vi "Single point scan V1.vi"() -> ()   [LabVIEW 2024]
uses:
  <vilib>/DAQmx/create/channels.llb/DAQmx Create Channel (AO-Voltage-Basic).vi
  <vilib>/DAQmx/miscellaneous.llb/DAQmx Fill In Error Info.vi
  <vilib>/DAQmx/configure/trigger.llb/DAQmx Start Trigger (None).vi
  <vilib>/DAQmx/configure/timing.llb/DAQmx Timing (Sample Clock).vi
  <vilib>/DAQmx/write.llb/DAQmx Write (Analog 1D DBL NChan 1Samp).vi
  <vilib>/DAQmx/read.llb/DAQmx Read (Analog 1D DBL 1Chan NSamp).vi
  <vilib>/DAQmx/create/channels.llb/DAQmx Create Channel (AI-Voltage-Basic).vi
  <vilib>/vision/driver/NI_Vision_Acquisition_Software.lvlib
panel:
  in  "Camera Name":refnum<k21> caption="IMAQdx Session"
  out "Image":T1(plugin-control)
  out "Filename Out":path
  in  "Filename":path=path "test.lvm"
  in  "Enable data file creation":bool=TRUE caption="Enable"
  out "output waveform":waveform(dbl)
  out "Waveform Graph":dbl[](graph)
  in  "start acquisition":bool
  in  "total samples":i32=1000
  in  "rate (Hz)":dbl=1000.0 format="%0.2f"
  in  "Y-axis":dbl(slide) scale=-10.0..10.0
  in  "X-axis":dbl(slide) scale=-10.0..10.0
  # "Data settings"
  # "Adjust Laser position"
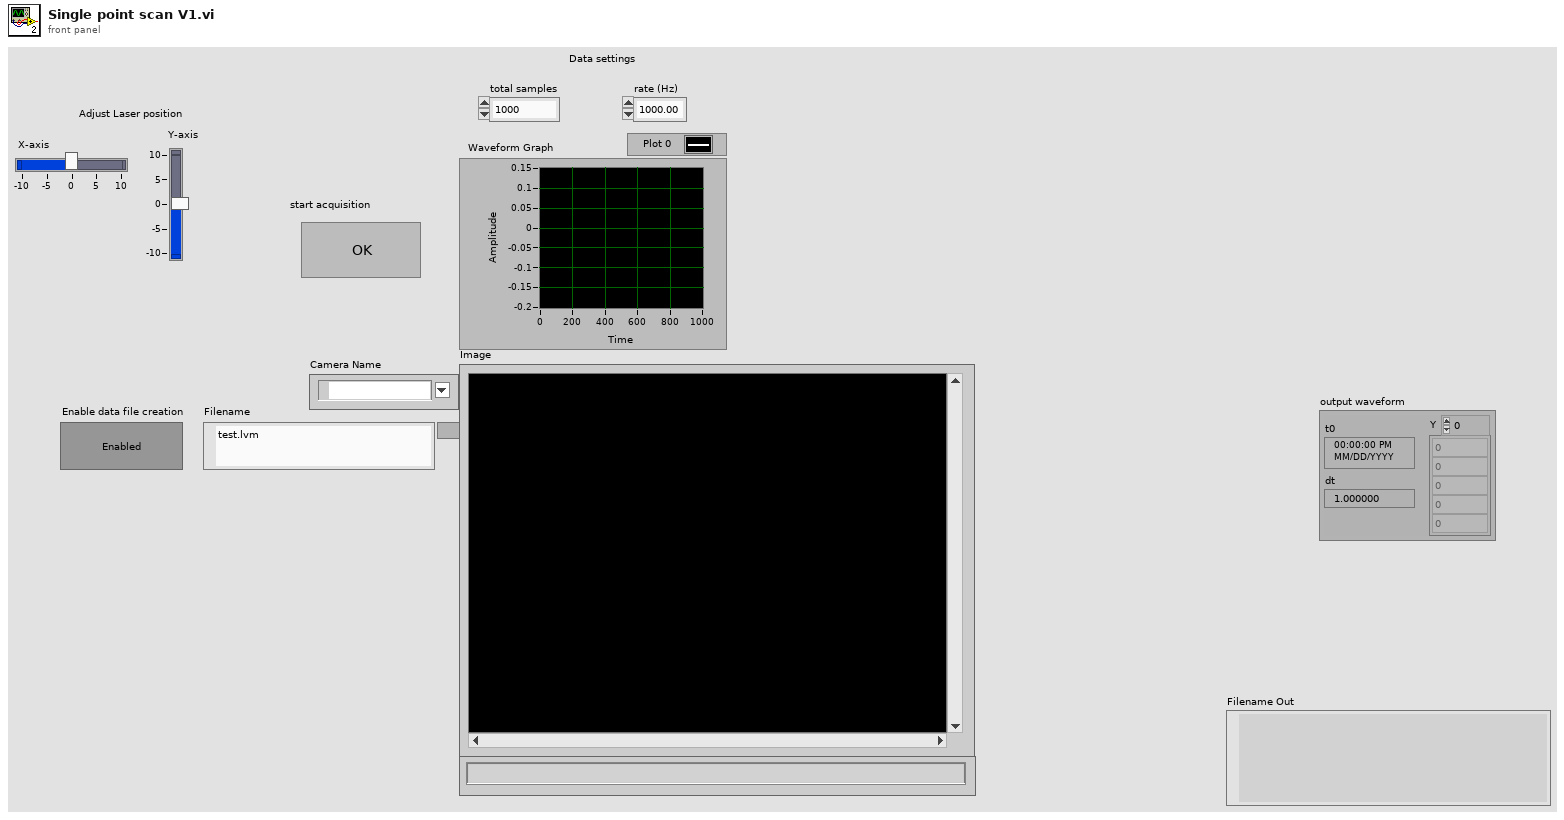
[diagram p1: front panel]
types:
  T1 = typedef "IMAQ Image.ctl" = refnum<image>
  T2 = typedef "IMAQdx.ctl" = refnum<k21>
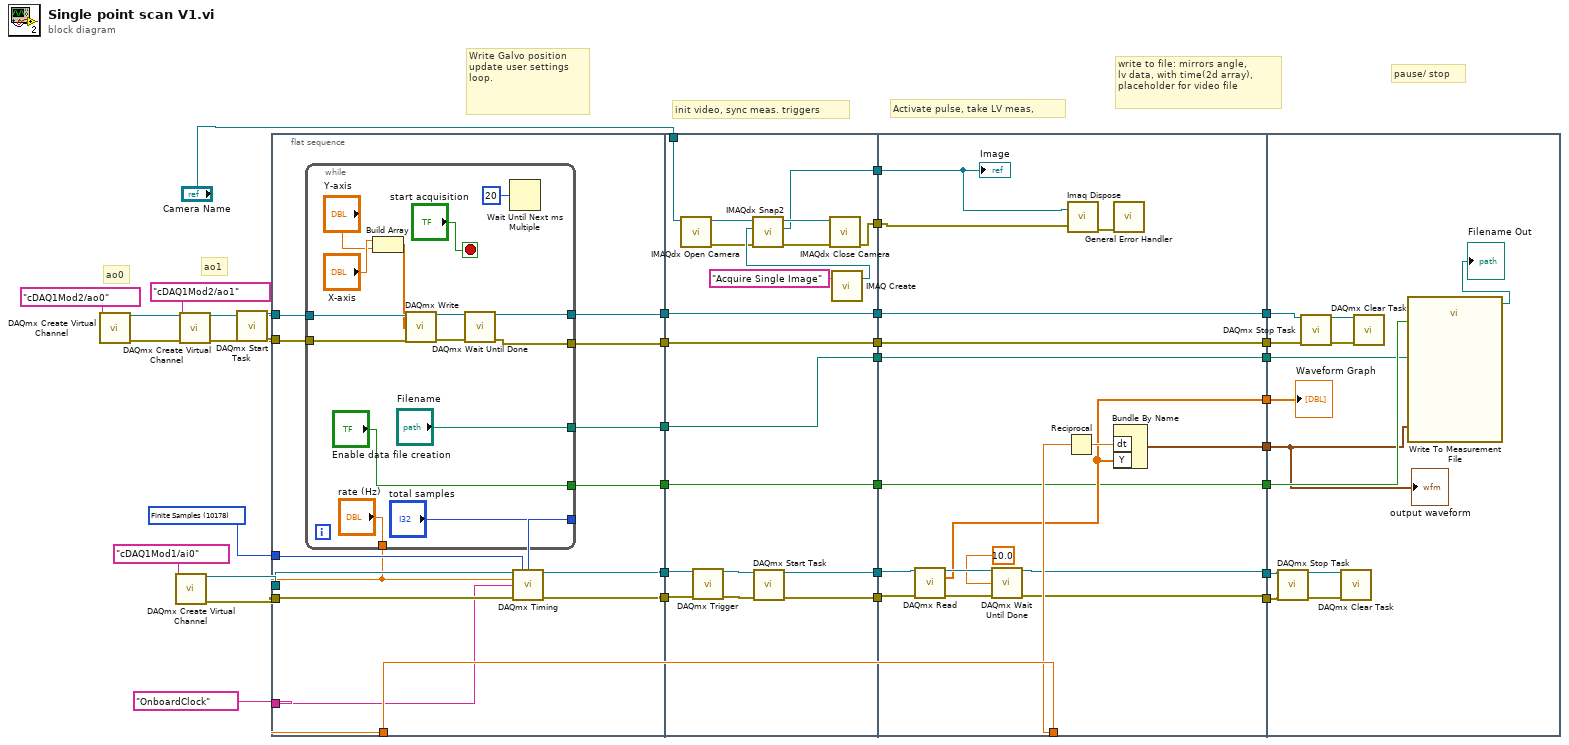
[diagram p0: block diagram]
diagram:
  w27 = 10178 items=["Finite Samples"=10178, "Continuous Samples"=10123, "Hardware Timed Single Point"=12522] ("sample mode")
  # "ao1"
  # "ao0"
  # "pause/ stop"
  # "write to file: mirrors angle, \nlv data, with time(2d array), \nplaceholder for video file"
  # "Activate pulse, take LV meas,"
  # "init video, sync meas. triggers"
  # "Write Galvo position\nupdate user settings loop."
  n1 = call-poly <vilib>:"DAQmx Create Virtual Channel.vi"("physical channels"=tag "cDAQ1Mod2/ao0") -> ("task out"=w37:refnum<k21>, "error out"=w36:errorcluster)  [unwired: 13 in]
  n2 = call-poly <vilib>:"DAQmx Create Virtual Channel.vi"("physical channels"=tag "cDAQ1Mod1/ai0") -> ("task out"=w28:refnum<k21>, "error out"=w26:errorcluster)  [unwired: 13 in]
  n3 = call-poly <vilib>:"DAQmx Create Virtual Channel.vi"("task in"=w37, "physical channels"=tag "cDAQ1Mod2/ao1", "error in"=w36) -> ("task out"=w4:refnum<k21>, "error out"=w3:errorcluster)  [unwired: 11 in]
  n4 = call <vilib>:"DAQmx Start Task.vi"("task/channels in"=w4, "error in"=w3) -> ("task out"=w2:refnum<k21>, "error out"=w1:errorcluster)  [unwired: 12 in]
  n5 = flat-sequence {
    tunnel: w2 -> [w51]
    tunnel: w1 -> [w50]
    tunnel: [w47] -> w32
    tunnel: [w46] -> w31
    tunnel: w28 -> [w49]
    tunnel: w27 -> [w45]
    tunnel: w26 -> [w48]
    tunnel: [w44] -> w25
    tunnel: tag "OnboardClock" ("source") -> [w42]
    tunnel: [w41] -> w21
    tunnel: [w40] -> w16
    tunnel: [w39] -> w11
    tunnel: [w38] -> w8
    tunnel: w32 -> [w83]
    tunnel: w31 -> [w82]
    tunnel: [w81] -> w30
    tunnel: [w80] -> w29
    tunnel: w21 -> [w79]
    tunnel: [w79] -> w20
    tunnel: [w78] -> w17
    tunnel: w16 -> [w78]
    tunnel: [w77] -> w12
    tunnel: w11 -> [w77]
    tunnel: [w76] -> w9
    tunnel: w8 -> [w76]
    tunnel: "Camera Name" -> [w70]
    tunnel: [w68] -> w7
    tunnel: [w67] -> w6
    tunnel: w30 -> [w103]
    tunnel: w29 -> [w102]
    tunnel: w25 -> [w100]
    tunnel: [w90] -> w23
    tunnel: [w89] -> w22
    tunnel: w20 -> [w96]
    tunnel: [w96] -> w19
    tunnel: [w95] -> w18
    tunnel: w17 -> [w95]
    tunnel: [w93] -> w15
    tunnel: [w94] -> w14
    tunnel: [w92] -> w13
    tunnel: w12 -> [w92]
    tunnel: [w91] -> w10
    tunnel: w9 -> [w91]
    tunnel: w7 -> [w86]
    tunnel: w6 -> [w87]
    tunnel: w23 -> [w116]
    tunnel: w22 -> [w115]
    tunnel: w19 -> [w110]
    tunnel: w18 -> [w109]
    tunnel: w15 -> [w107]
    tunnel: w14 -> [w105]
    tunnel: w13 -> [w108]
    tunnel: w10 -> [w106]
    frame #0 {
      n6 = while {
        tunnel: w51 -> [w65]
        tunnel: w50 -> [w64]
        tunnel: ["rate (Hz)"] -> w44
        tunnel: ["total samples"] -> w43
        tunnel: [w58] -> w41
        tunnel: [w57] -> w40
        tunnel: ["Enable data file creation"] -> w39
        tunnel: ["Filename"] -> w38
        stop <- "start acquisition" stop-if-true
        n7 = Build Array("X-axis", "Y-axis") -> (w63:dbl[])
        n8 = call-poly <vilib>:"DAQmx Write.vi"("task/channels in"=w65, "data"=w63, "error in"=w64) -> ("task out"=w62:refnum<k21>, "error out"=w61:errorcluster)  [unwired: 10 in, 1 out]
        n9 = call <vilib>:"DAQmx Wait Until Done.vi"("task/channels in"=w62, "error in"=w61) -> ("task out"=w58:refnum<k21>, "error out"=w57:errorcluster)  [unwired: 12 in]
        n10 = Wait Until Next ms Multiple(millisecond multiple=u32 20) -> ()  [unwired: 1 out]
      }
      n11 = call-poly <vilib>:"DAQmx Timing.vi"("task/channels in"=w49, "sample mode"=w45, "samples per channel"=w43, "rate"=w44, "source"=w42, "error in"=w48) -> ("task out"=w47:refnum<k21>, "error out"=w46:errorcluster)  [unwired: 8 in]
    }
    frame #1 {
      n12 = call <vilib>:"IMAQdx Open Camera.vi"("Session In"=w70) -> ("error out"=w74:errorcluster, "Session Out"=w72:T2)  [unwired: 2 in, 7 out]
      n13 = call-poly <vilib>:"DAQmx Trigger.vi"("task/channels in"=w83, "error in"=w82) -> ("task out"=w85:refnum<k21>, "error out"=w84:errorcluster)  [unwired: 12 in]
      n14 = call <vilib>:"DAQmx Start Task.vi"("task/channels in"=w85, "error in"=w84) -> ("task out"=w81:refnum<k21>, "error out"=w80:errorcluster)  [unwired: 12 in]
      n15 = call "IMAQ Create"("Image Name"="Acquire Single Image") -> ("New Image"=w75:T1)  [unwired: 3 in, 2 out]
      n16 = call <vilib>:"IMAQdx Snap2.vi"("error in"=w74, "Image In"=w75, "Session In"=w72) -> ("error out"=w73:errorcluster, "Image Out"=w68:T1, "Session Out"=w71:T2)  [unwired: 6 in]
      n17 = call <vilib>:"IMAQdx Close Camera.vi"("error in"=w73, "Session In"=w71) -> ("error out"=w67:errorcluster)  [unwired: 9 out]
    }
    frame #2 {
      n18 = call-poly <vilib>:"DAQmx Read.vi"("task/channels in"=w103, "error in"=w102) -> ("task out"=w99:refnum<k21>, "data"=w93:dbl[], "error out"=w98:errorcluster)  [unwired: 11 in]
      n19 = call <vilib>:"DAQmx Wait Until Done.vi"("task/channels in"=w99, "timeout (sec)"=10.0, "error in"=w98) -> ("task out"=w90:refnum<k21>, "error out"=w89:errorcluster)  [unwired: 11 in]
      n20 = Reciprocal(x=w100) -> (1/x=w101:dbl)
      n21 = call "Imaq Dispose"("Image"=w86, "error in (no error)"=w87) -> ("error out"=w88:errorcluster)  [unwired: 4 in]
      n22 = call <vilib>:"General Error Handler.vi"("error in (no error)"=w88) -> ()  [unwired: 2 in, 13 out]
      n23 = Bundle By Name("dt"=w101, "Y"=w93) -> (w94:waveform(dbl))  [unwired: 1 in]
      "Image" <- w86
    }
    frame #3 {
      n24 = call <vilib>:"DAQmx Stop Task.vi"("task/channels in"=w116, "error in"=w115) -> ("task out"=w114:refnum<k21>, "error out"=w113:errorcluster)  [unwired: 12 in]
      n25 = call <vilib>:"DAQmx Stop Task.vi"("task/channels in"=w110, "error in"=w109) -> ("task out"=w112:refnum<k21>, "error out"=w111:errorcluster)  [unwired: 12 in]
      n26 = call <vilib>:"DAQmx Clear Task.vi"("task in"=w114, "error in"=w113) -> ()  [unwired: 13 in, 1 out]
      n27 = call <vilib>:"DAQmx Clear Task.vi"("task in"=w112, "error in"=w111) -> ()  [unwired: 13 in, 1 out]
      n28 = call "Write To Measurement File"("Signals"=w105, "Enable"=w108, "Filename"=w106) -> ("Filename Out"=→"Filename Out":path)  [unwired: 14 in, 2 out]
      "Waveform Graph" <- w107
      "output waveform" <- w105
    }
  }
